vi "Charging_Mean IPG State.vi"(7 "Samples (10)":i32=10, 8 "error in":errorcluster, 9 "Abort Threshold (42 C)":dbl=42.0 format="%5.5f", 10 "Critical Threshold (41 C)":dbl=41.0 format="%5.5f", 11 "Warning Threshold (40 C)":dbl=40.0 format="%5.5f") -> (0 "error out":errorcluster, 1 "IPG_ReceivedLevel":dbl=nan, 2 "xPG Temperature Level":dbl=nan, 3 "ChargingState":string, 5 "Compensated Temperature (C)":dbl=nan format="%.3f")   [LabVIEW 2010]
uses:
  <vilib>/Analysis/NI_AALBase.lvlib
panel:
  out "Log":dbl[](array[numeric]) format="%.2f"
  # "GEN CALS"
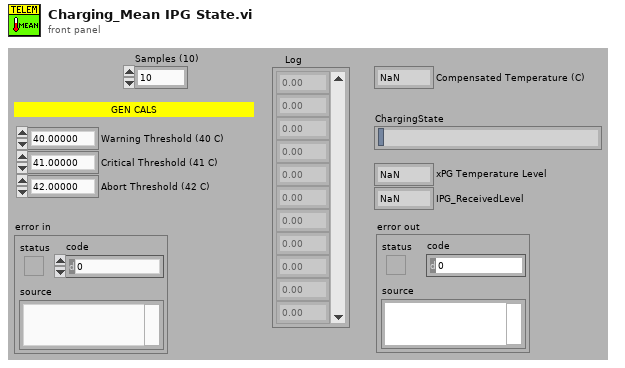
[diagram p1: front panel]
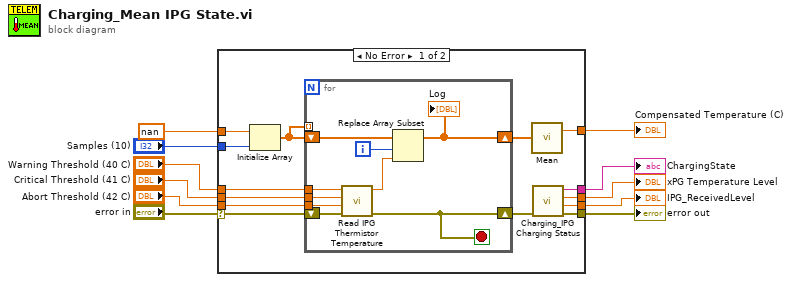
[diagram p0: block diagram]
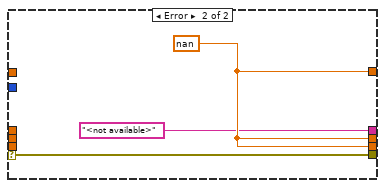
[diagram p2: hidden frame]
diagram:
  n1 = case shown="No Error" "error in" {
    selector: "error in" -> [w16 w37]
    tunnel: [w25 w36] -> w11
    tunnel: [w24 w36] -> w10
    tunnel: [w22 "<not available>" ("ChargingState")] -> w9
    tunnel: "Abort Threshold (42 C)" -> [w21 _]
    tunnel: "Critical Threshold (41 C)" -> [w20 _]
    tunnel: "Warning Threshold (40 C)" -> [w19 _]
    tunnel: [w17 w36] -> w5
    tunnel: "Samples (10)" -> [w14 _]
    tunnel: [w15 w37] -> w2
    tunnel: nan ("element") -> [w13 _]
    frame No Error {
      n2 = Initialize Array(w13, w14) -> (w12:dbl[])
      n3 = for {
        shift-right: [w30] -> w23
        shift-left: w16 -> [w34]
        tunnel: w21 -> [w33]
        tunnel: w20 -> [w32]
        tunnel: w19 -> [w31]
        shift-right: [w28] -> w18
        shift-left: w12 -> [w29]
        tunnel: w12 -> [_] mode=indexing
        i -> [w26]
        stop <- w30 stop-if-true
        n4 = call "Read IPG Thermistor Temperature.vi"("error in"=w34, "Abort Threshold (42 C)"=w33, "Critical Threshold (41 C)"=w32, "Warning Threshold (40 C)"=w31) -> ("error out"=w30:errorcluster, "Compensated Temperature (C)"=w27:dbl)  [unwired: 4 in, 2 out]
        n5 = Replace Array Subset "Replace Array Subset"(array=w29, new element=w27, index=w26) -> (w28:dbl[])
        "Log" <- w28
      }
      n6 = call <vilib>:"Mean.vi"("X"=w18) -> ("mean"=w17:dbl)  [unwired: 1 out]
      n7 = call "Charging_IPG Charging Status.vi"("error in"=w23) -> ("error out"=w15:errorcluster, "IPG_ReceivedLevel"=w24:dbl, "TemperatureLevel"=w25:dbl, "ChargingState"=w22:string)  [unwired: 7 in]
    }
    frame Error {
      w36 = nan ("mean")
    }
  }
  "xPG Temperature Level" <- w11
  "IPG_ReceivedLevel" <- w10
  "Compensated Temperature (C)" <- w5
  "ChargingState" <- w9
  "error out" <- w2
